vi "LcWebView_example_2.vi"() -> ()   [LabVIEW 2018, in "LcWebView.lvclass"]
uses:
  LcWebView.lvclass
  D:/GitProjects/Public/GitHub/LcWebView/data/Microsoft.Web.WebView2.WinForms.dll
  data/Microsoft.Web.WebView2.WinForms.dll
panel:
  out "Javascript result":string
  out "Initialise Loops":i32
  out "Status Message":string
  out "Status":i32(ring) items=["Created", "WaitingForActivation", "WaitingToRun", "Running", "WaitingForChildrenToComplete", "RanToCompletion", "Canceled", "Faulted"]
  out "Error Out":errorcluster
  in  "stop":bool
  in  "Web":refnum<k24>(container)
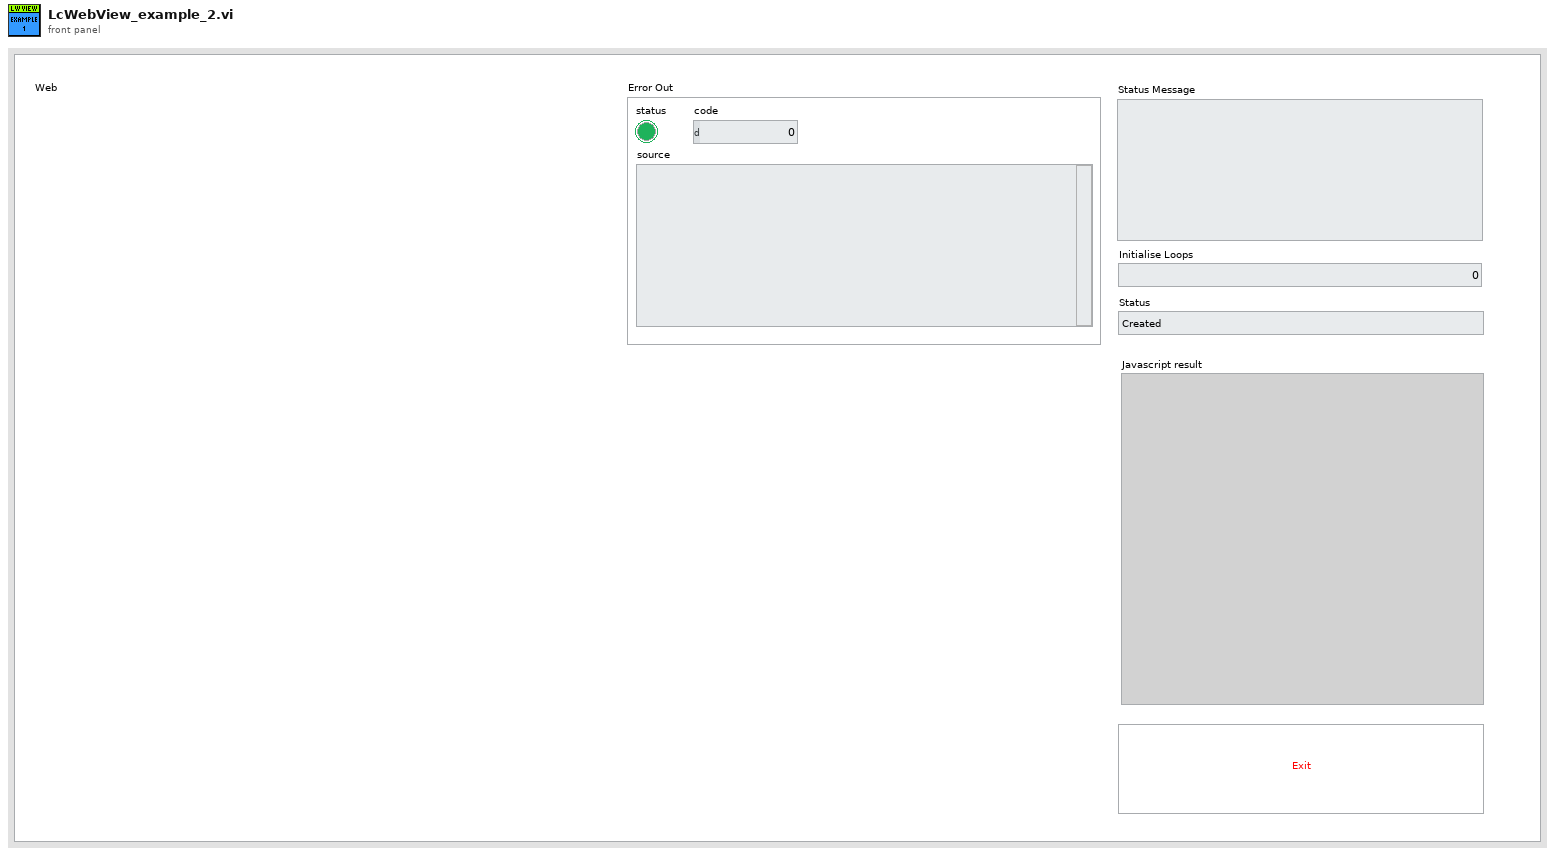
[diagram p1: front panel]
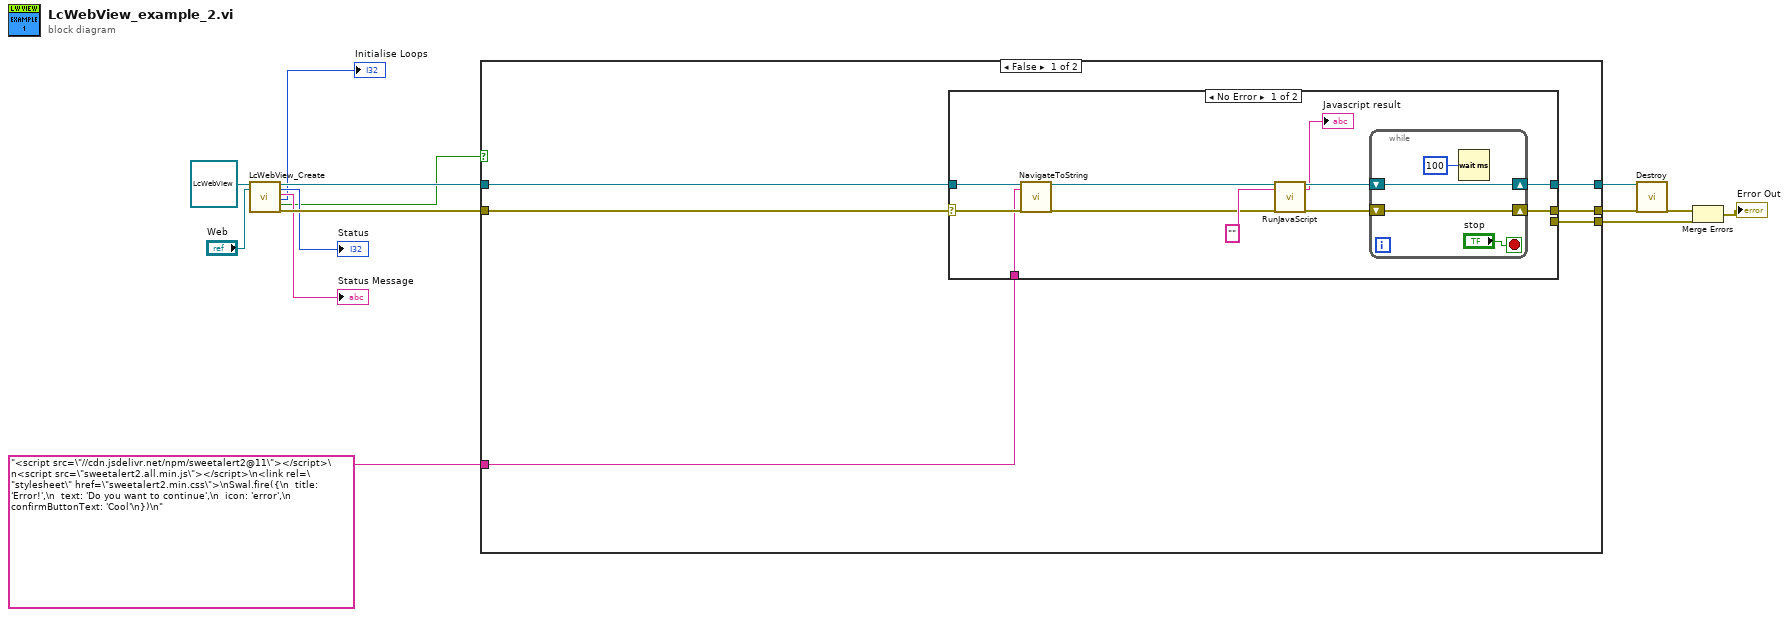
[diagram p0: block diagram]
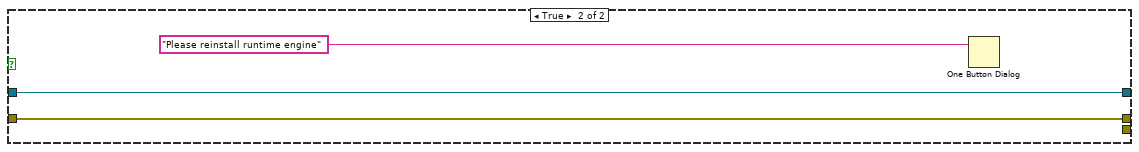
[diagram p3: hidden frame]
diagram:
  n1 = call "LcWebView_Create.vi"("reference in"=refnum<class "LcWebView.lvclass"> refnum, "Webview container"="Web") -> ("reference out"=w12:refnum<class "LcWebView.lvclass">, "Status"=→"Status":i32, "Status Message"=→"Status Message":string, "Initialise Loops"=→"Initialise Loops":i32, "Reinstall Runtime"=w3:bool, "Error Out"=w11:errorcluster)  [unwired: 10 in, 2 out]
  n2 = case shown="False" w3 {
    tunnel: w12 -> [w20 w40]
    tunnel: w11 -> [w19 w39]
    tunnel: [w18 w40] -> w10
    tunnel: [w17 w39] -> w9
    tunnel: [w16 _] -> w4
    tunnel: "<script src=\"//cdn.jsdelivr.net/npm/sweetalert2@11\"></script>\n<script src=\"sweetalert2.all.min.js\"></script>\n<link rel=\"stylesheet\" href=\"sweetalert2.min.css\">\nSwal.fire({\n  title: 'Error!',\n  text: 'Do you want to continue',\n  icon: 'error',\n  confirmButtonText: 'Cool'\n})\n" ("HTML Content") -> [w15 _]
    frame False {
      n3 = case shown="No Error" w19 {
        selector: w19 -> [w22 w36]
        tunnel: w20 -> [w23 w37]
        tunnel: [w31 w37] -> w18
        tunnel: [w30 _] -> w17
        tunnel: [_ w36] -> w16
        tunnel: w15 -> [w21 _]
        frame No Error {
          n4 = call-dynamic "NavigateToString.vi"("reference in"=w23, "HTML Content"=w21, "Error In"=w22) -> ("reference out"=w25:refnum<class "LcWebView.lvclass">, "Error Out"=w24:errorcluster)  [unwired: 14 in, 1 out]
          n5 = call-dynamic "RunJavaScript.vi"("reference in"=w25, "Java Script Function"="", "Error In"=w24) -> ("reference out"=w29:refnum<class "LcWebView.lvclass">, "Result"=→"Javascript result":string, "Error Out"=w28:errorcluster)  [unwired: 13 in, 1 out]
          n6 = while {
            shift-right: [w34] -> w31
            shift-left: w29 -> [w34]
            shift-right: [w33] -> w30
            shift-left: w28 -> [w33]
            stop <- "stop" stop-if-true
            n7 = Wait (ms)(milliseconds to wait=u32 100) -> ()  [unwired: 1 out]
          }
        }
        frame Error {
        }
      }
    }
    frame True {
      n8 = One Button Dialog(message="Please reinstall runtime engine") -> ()  [unwired: 1 in, 1 out]
    }
  }
  n9 = call-dynamic "Destroy.vi"("reference in"=w10, "Error In"=w9) -> ("Error Out"=w8:errorcluster)  [unwired: 16 in, 1 out]
  n10 = Merge Errors(w8, w4) -> (→"Error Out":errorcluster)
